vi "TS-70.vi"() -> ()   [LabVIEW 2018]
uses:
  <vilib>/DAQmx/write.llb/DAQmx Write (Analog 1D DBL NChan 1Samp).vi
  <vilib>/DAQmx/write.llb/DAQmx Write (Digital 1D Bool NChan 1Samp 1Line).vi
  <vilib>/DAQmx/read.llb/DAQmx Read (Analog 1D DBL NChan 1Samp).vi
  <vilib>/DAQmx/read.llb/DAQmx Read (Counter 1D DBL 1Chan NSamp).vi
  <vilib>/DAQmx/read.llb/DAQmx Read (Analog 1D Wfm NChan NSamp).vi
  <vilib>/DAQmx/write.llb/DAQmx Write (Analog DBL 1Chan 1Samp).vi
  <vilib>/DAQmx/create/channels.llb/DAQmx Create Channel (AI-Voltage-Basic).vi
  <vilib>/DAQmx/create/channels.llb/DAQmx Create Channel (CI-Frequency).vi
  <vilib>/DAQmx/configure/timing.llb/DAQmx Timing (Implicit).vi
  <vilib>/DAQmx/create/channels.llb/DAQmx Create Channel (AI-Temperature-Thermocouple).vi
  <vilib>/DAQmx/create/channels.llb/DAQmx Create Channel (DO-Digital Output).vi
  <vilib>/DAQmx/miscellaneous.llb/DAQmx Fill In Error Info.vi
  <vilib>/DAQmx/create/channels.llb/DAQmx Create Channel (AO-Voltage-Basic).vi
  <vilib>/DAQmx/create/channels.llb/DAQmx Create Channel (AI-Current-Basic).vi
  <vilib>/ptbypt/NI_PtbyPt.lvlib
  <resource>/objmgr/daqmx.rc
panel:
  out "Digital Out Errors":errorcluster
  in  "Sample Data":bool
  in  "?":T1(tab)
  out "Case Temp":i32
  out "Inlet Temp":i16
  out "RPM":i16 format="%2.0f"
  out "DisGPMCal":dbl caption="Dis GPM" format="%2.0f"
  out "CaseGPM":dbl caption="Case GPM" format="%2.0f"
  out "PSI Case":dbl caption="Case PSI" format="%2.0f"
  out "PSI In":dbl caption="Inlet PSI" format="%2.0f"
  out "PSI Discharge":dbl caption="Dis PSI" format="%2.0f"
  out "Amps C - Main":dbl caption="Amps C" format="%#.2g"
  out "Amps B - Main":dbl caption="Amps B" format="%#.2g"
  out "Amps A - Main":dbl caption="Amps A" format="%#.2g"
  out "C Volts - Main":i32 caption="VAC C"
  out "B Volts - Main":i32 caption="VAC B"
  out "A Volts - Main":i32 caption="VAC A"
  out "AC Hz":i32 caption="Hz"
  in  "Sample Rate (ms)":u32=5
  out "Waveform Chart":waveform(dbl)[](graph)
  out "Output\nVoltage - Main":dbl(knob) caption="Regulator VDC" scale=0.0..10.0
  out "Amps C - Tank":u8(slide) scale=0.0..100.0
  out "Amps B - Tank":u8(slide) scale=0.0..100.0
  out "Amps A - Tank":u8(slide) scale=0.0..100.0
  out "C Volts - Ammeter":dbl caption="C VAC" format="%#_3f"
  out "B Volts - Ammeter":dbl caption="B VAC" format="%#_3f"
  out "A Volts - Ammeter":dbl caption="A VAC" format="%#_3f"
  out "AC Hz 2":dbl caption="Hz" format="%#_3f"
  out "Amps C - Ammeters":dbl caption="C Phase" format="%#.2g"
  out "Amps B - Ammeters":dbl caption="B Phase" format="%#.2g"
  out "Amps A - Ammeters":dbl caption="A Phase" format="%#.2g"
  in  "PS 1 On/Off":bool
  in  "PS 2 On/Off":bool
  out "PS1 Amps":dbl format="%#.2f"
  out "PS1 Output Gauge":dbl(knob) scale=0.0..36.0
  out "PS1 Output":dbl format="%.1f"
  in  "PS1 Scale":dbl=10.25
  in  "PS1 Offset":dbl
  out "PS1 Desired":dbl format="%.1f"
  in  "PS1 Control":dbl(slide)=28.0 min=0.0 max=36.0 step=0.5 scale=0.0..36.0
  out "PS1 Control VDC":dbl
  in  "Output Scale":dbl=1.0
  out "PS2 Amps":dbl format="%#.2f"
  out "PS2 Outpug Gauge":dbl(knob) scale=0.0..36.0
  out "PS2 Output":dbl format="%.1f"
  in  "PS2 Scale":dbl=10.07
  in  "PS2 Offset":dbl
  out "PS2 Desired":dbl format="%.1f"
  in  "PS2 Control":dbl(slide)=28.0 min=0.0 max=36.0 step=0.5 scale=0.0..36.0
  out "PS2 Control VDC":dbl
  in  "Output Scale 2":dbl=1.0
  out "Temp Setting\nError":bool
  out "Output\nVoltage - Temp":dbl(knob) scale=0.0..10.0
  in  "Low Temp":i16
  in  "High Temp":i16
  out "Case Temp 2":i16(slide) scale=-25.0..250.0
  out "Inlet Temp 2":i16(slide) scale=-25.0..250.0
  in  "Relay 4":bool
  in  "Timed Relay":bool
  out "Boolean":bool
  in  "Off Time":dbl=1.0
  in  "On Time":dbl=2.0
  in  "RPM Offset":dbl format="%#_13g"
  in  "RPM Scale":dbl=1.0 format="%#_13g"
  out "RPM":i16 caption="Indicated"
  in  "CaseGPM Offset":dbl format="%#_13g"
  in  "CaseGPM Scale":dbl=1.0 format="%#_13g"
  out "CaseGPMCal":dbl caption="Indicated"
  in  "DisGPM Offset":dbl format="%#_13g"
  in  "DisGPM Scale":dbl=10.0 format="%#_13g"
  out "DisGPM":dbl caption="Indicated"
  in  "CasePSI Offset":dbl format="%#_13g"
  in  "CasePSI Scale":dbl=200.0 format="%#_13g"
  out "CasePSI":dbl caption="Indicated"
  in  "InPSI Offset":dbl format="%#_13g"
  in  "InPSI Scale":dbl=100.0 format="%#_13g"
  out "InPSI Ind":dbl caption="Indicated"
  in  "DisPSI Offset":dbl format="%#_13g"
  in  "DisPSI Scale":dbl=1000.0 format="%#_13g"
  out "DisPSI - Calibration":dbl caption="Indicated"
  out "AC Freq Ind":dbl caption="Indicated"
  in  "AC Freq Offset":dbl=10.0 caption="Offset" format="%#_13g"
  in  "AC Freq Scale":dbl=100.0 caption="Scale" format="%#_13g"
  out "A VAC Ind":dbl caption="Indicated"
  in  "VAC Offset A":dbl caption="Offset" format="%#_13g"
  in  "VAC Scale A":dbl=50.0 caption="Scale" format="%#_13g"
  out "B Volts - Calibration":dbl caption="Indicated"
  in  "Amp Offset C":dbl format="%#_13g"
  in  "Amp Offset B":dbl format="%#_13g"
  in  "Amp Offset A":dbl format="%#_13g"
  in  "Amp Scale C":dbl=9.88 format="%#_13g"
  in  "Amp Scale B":dbl=9.88 format="%#_13g"
  in  "Amp Scale A":dbl=9.88 format="%#_13g"
  in  "VAC Scale B":dbl=50.0 caption="Scale" format="%#_13g"
  in  "VAC Offset B":dbl caption="Offset" format="%#_13g"
  in  "VAC Offset C":dbl caption="Offset" format="%#_13g"
  in  "VAC Scale C":dbl=50.0 caption="Scale" format="%#_13g"
  out "C Volts - Calibration":dbl caption="Indicated"
  out "Amps A - Calibration":dbl caption="Indicated"
  out "Amps B - Calibration":dbl caption="Indicated"
  out "Amps C - Calibration":dbl caption="Indicated"
  out "error out":errorcluster
  out "Analog Out Errors":errorcluster
  # "AC Frequency"
  # "A Phase VAC"
  # "B Phase VAC"
  # "C Phase VAC"
  # "A Phase Amps"
  # "B Phase Amps"
  # "C Phase Amps"
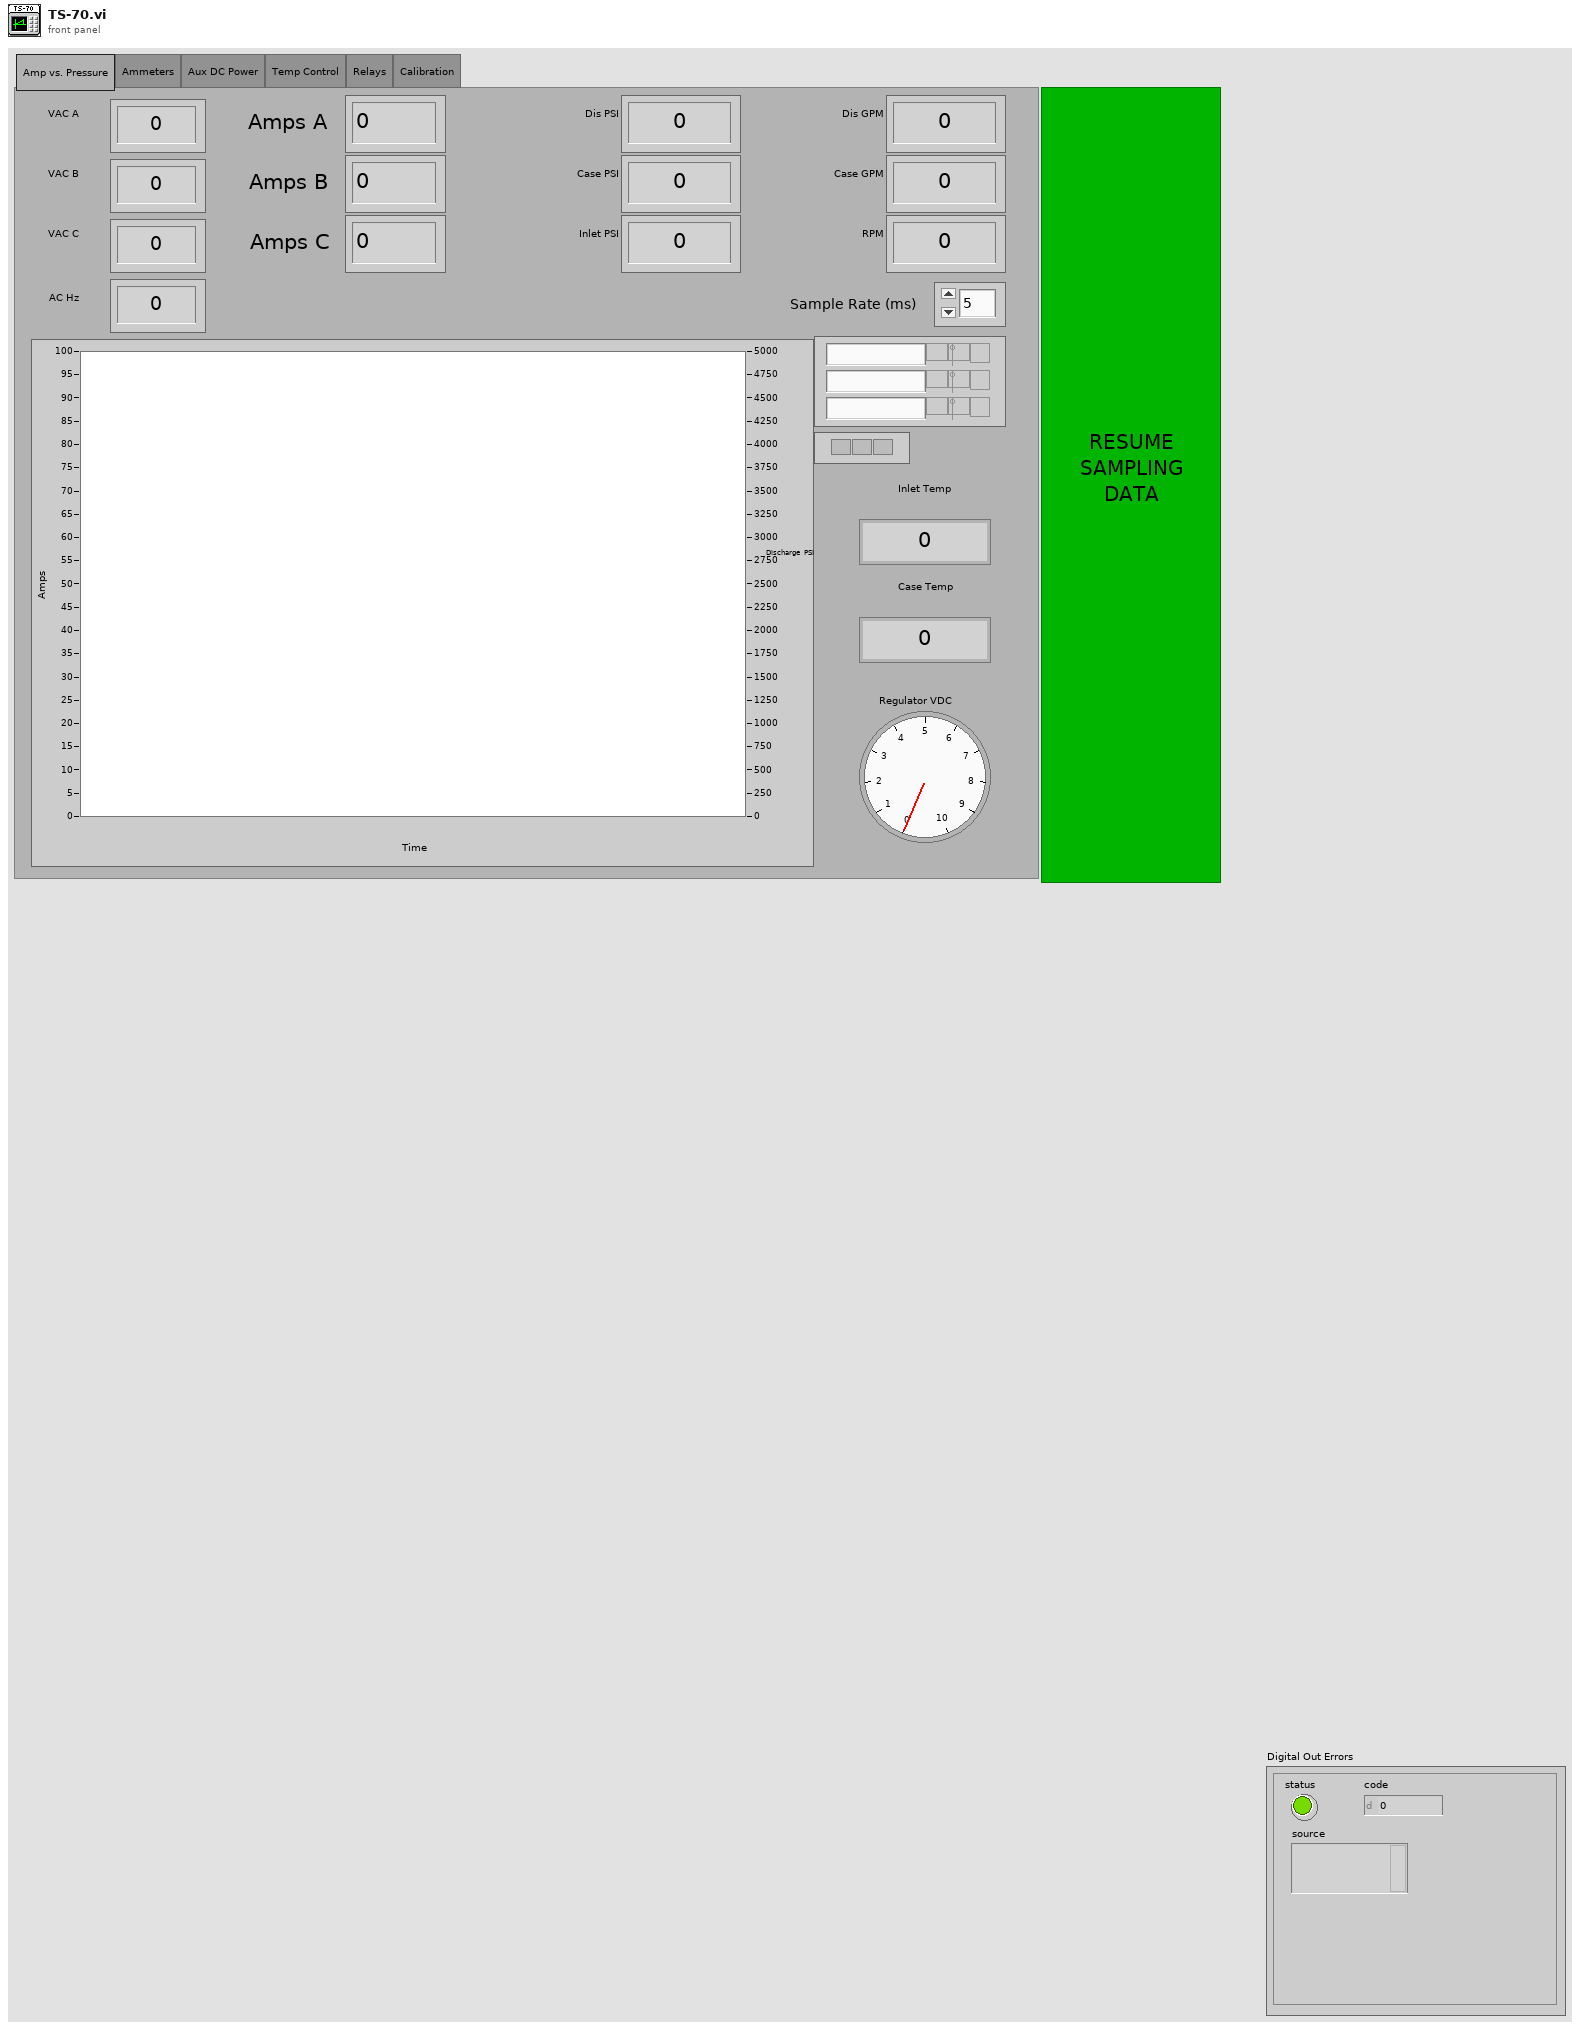
[diagram p1: front panel]
types:
  T1 = enum32{"Amp vs. Pressure", "Ammeters", "Aux DC Power", "Temp Control", "Relays", "Calibration"}
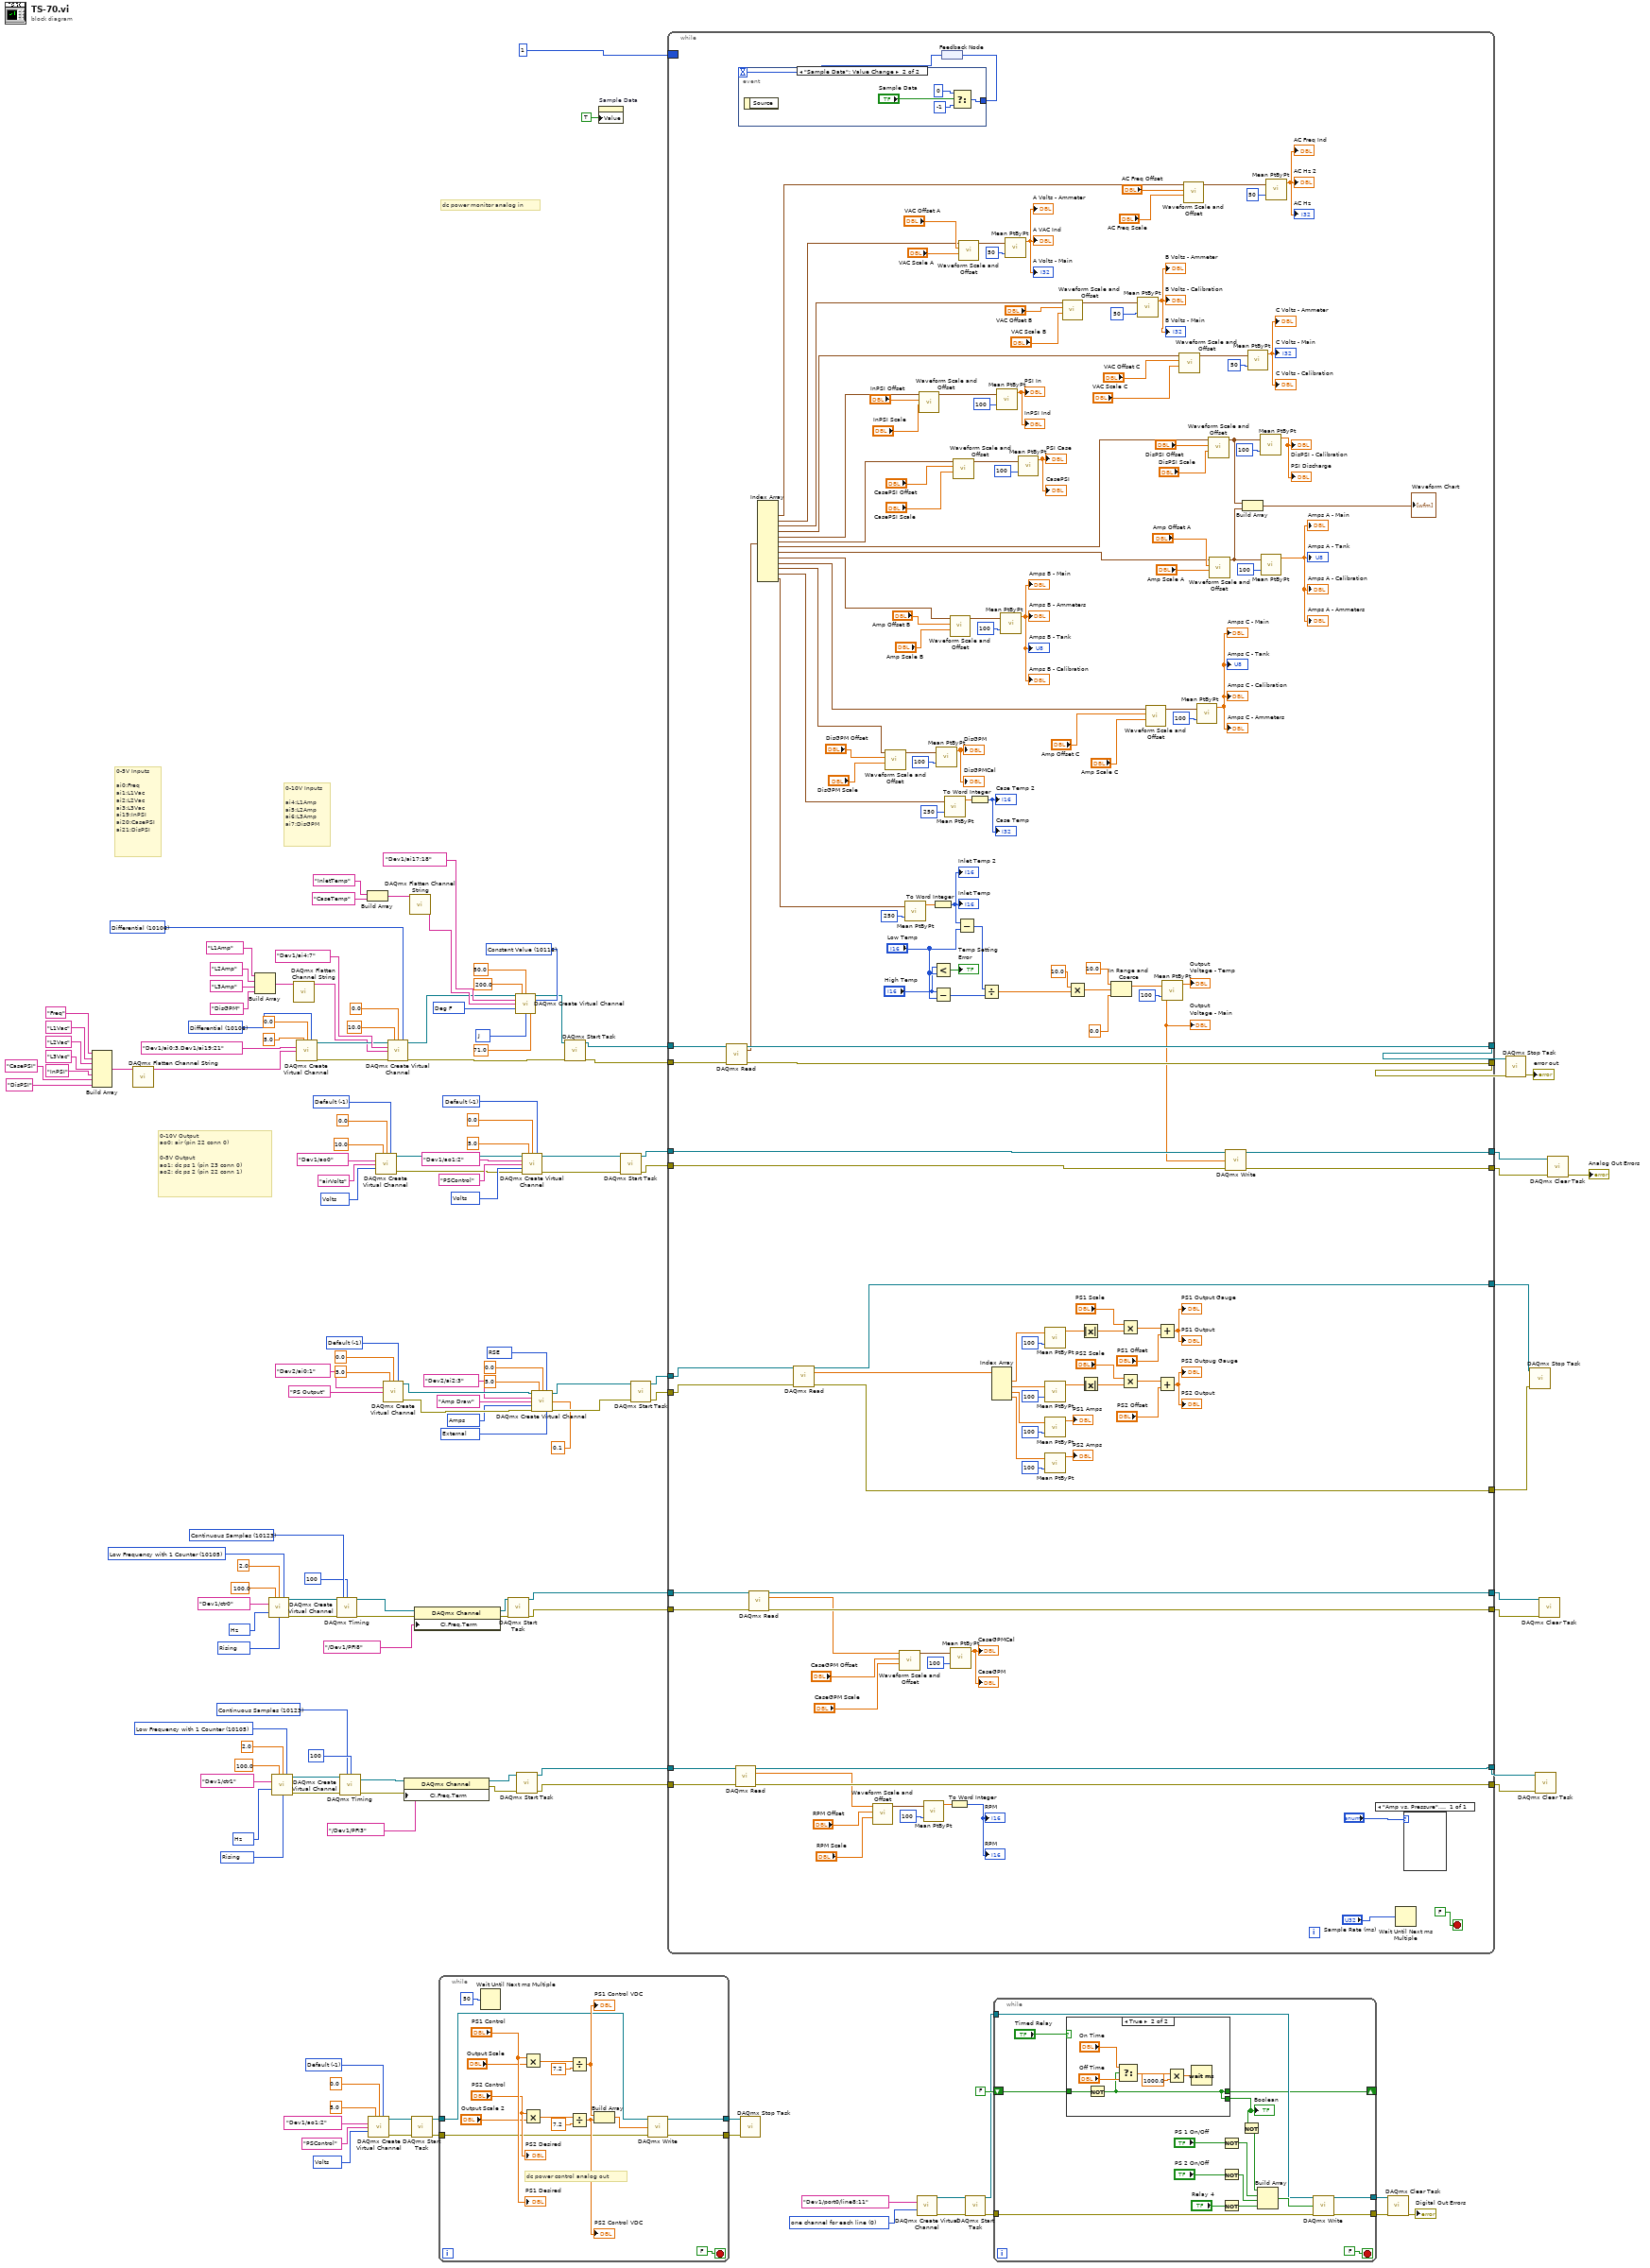
[diagram p0: block diagram]
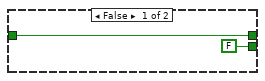
[diagram p2: hidden frame]
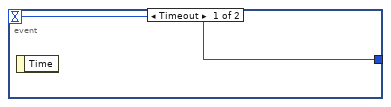
[diagram p3: hidden frame]
diagram:
  w5 = -1 items=["Default"=-1, "RSE"=10083, "Differential"=10106, "Pseudodifferential"=12529] ("output terminal configuration")
  w10 = 10348 items=["Volts"=10348, "From Custom Scale"=10065] ("units")
  w17 = 10167 items=["default"=-1, "Internal"=10200, "External"=10167] ("shunt resistor location")
  w19 = 10342 items=["Amps"=10342, "From Custom Scale"=10065] ("units")
  w22 = 10083 items=["default"=-1, "RSE"=10083, "NRSE"=10078, "Differential"=10106, "Pseudodifferential"=12529] ("input terminal configuration")
  w31 = -1 items=["Default"=-1, "RSE"=10083, "NRSE"=10078, "Differential"=10106, "Pseudodifferential"=12529] ("input terminal configuration")
  w38 = -1 items=["Default"=-1, "RSE"=10083, "Differential"=10106, "Pseudodifferential"=12529] ("output terminal configuration")
  w43 = 10348 items=["Volts"=10348, "From Custom Scale"=10065] ("units")
  w49 = -1 items=["Default"=-1, "RSE"=10083, "Differential"=10106, "Pseudodifferential"=12529] ("output terminal configuration")
  w54 = 10348 items=["Volts"=10348, "From Custom Scale"=10065] ("units")
  w61 = 0 items=["one channel for each line", "one channel for all lines"] ("line grouping")
  w68 = 10144 items=["Deg C"=10143, "Deg F"=10144, "Kelvins"=10325, "Deg R"=10145, "From Custom Scale"=10065] ("units")
  w69 = 10116 items=["Built-In"=10200, "Constant Value"=10116, "Channel"=10113] ("cjc source")
  w77 = 10072 items=["J"=10072, "K"=10073, "N"=10077, "R"=10082, "S"=10085, "T"=10086, "B"=10047, "E"=10055] ("thermocouple type")
  w92 = 10105 items=["Low Frequency with 1 Counter"=10105, "High Frequency with 2 Counters"=10157, "Large Range with 2 Counters"=10205, "Dynamic Averaging"=16065] ("measurement method")
  w91 = 10280 items=["Rising"=10280, "Falling"=10171] ("starting edge")
  w90 = 10373 items=["Hz"=10373, "Ticks"=10304, "From Custom Scale"=10065] ("units")
  w88 = 10123 items=["Finite Samples"=10178, "Continuous Samples"=10123, "Hardware Timed Single Point"=12522] ("sample mode")
  w107 = 10105 items=["Low Frequency with 1 Counter"=10105, "High Frequency with 2 Counters"=10157, "Large Range with 2 Counters"=10205, "Dynamic Averaging"=16065] ("measurement method")
  w108 = 10280 items=["Rising"=10280, "Falling"=10171] ("starting edge")
  w109 = 10373 items=["Hz"=10373, "Ticks"=10304, "From Custom Scale"=10065] ("units")
  w111 = 10123 items=["Finite Samples"=10178, "Continuous Samples"=10123, "Hardware Timed Single Point"=12522] ("sample mode")
  w142 = 10106 items=["default"=-1, "RSE"=10083, "NRSE"=10078, "Differential"=10106, "Pseudodifferential"=12529] ("input terminal configuration")
  w145 = 10106 items=["default"=-1, "RSE"=10083, "NRSE"=10078, "Differential"=10106, "Pseudodifferential"=12529] ("input terminal configuration")
  # "dc power monitor analog in"
  # "0-10V Output\nao0: air (pin 22 conn 0)\n\n0-5V Output\nao1: dc ps 1 (pin 23 conn 0)\nao2: dc ps 2 (pin 22 conn 1)"
  # "0-10V Inputs\n\nai4:L1Amp\nai5:L2Amp\nai6:L3Amp\nai7:DisGPM"
  # "0-5V Inputs\n\nai0:Freq\nai1:L1Vac\nai2:L2Vac\nai3:L3Vac\nai19:InPSI\nai20:CasePSI\nai21:DisPSI"
  n1 = Build Array("Freq", "L1Vac", "L2Vac", "L3Vac", "InPSI" ("element"), "CasePSI", "DisPSI") -> (w128:string[])
  n2 = call <vilib>:"DAQmx Flatten Channel String.vi"("names in"=w128) -> ("names out"=w127:string)  [unwired: 13 in, 1 out]
  n3 = Build Array("L1Amp", "L2Amp", "L3Amp", "DisGPM" ("element")) -> (w125:string[])
  n4 = call-poly <vilib>:"DAQmx Create Virtual Channel.vi"("maximum value"=100.0, "minimum value"=2.0, "measurement method"=w107, "counter"=tag "Dev1/ctr0", "units"=w109, "starting edge"=w108) -> ("task out"=w112:refnum<k21>, "error out"=w113:errorcluster)  [unwired: 8 in]
  n5 = call-poly <vilib>:"DAQmx Create Virtual Channel.vi"("maximum value"=100.0, "minimum value"=2.0, "measurement method"=w92, "counter"=tag "Dev1/ctr1", "units"=w90, "starting edge"=w91) -> ("task out"=w87:refnum<k21>, "error out"=w86:errorcluster)  [unwired: 8 in]
  n6 = call <vilib>:"DAQmx Flatten Channel String.vi"("names in"=w125) -> ("names out"=w121:string)  [unwired: 13 in, 1 out]
  n7 = call-poly <vilib>:"DAQmx Create Virtual Channel.vi"("maximum value"=5.0, "minimum value"=0.0, "input terminal configuration"=w145, "physical channels"=tag "Dev1/ai0:3,Dev1/ai19:21", "name to assign"=w127) -> ("task out"=w138:refnum<k21>, "error out"=w139:errorcluster)  [unwired: 9 in]
  n8 = call-poly <vilib>:"DAQmx Timing.vi"("task/channels in"=w112, "sample mode"=w111, "samples per channel"=100, "error in"=w113) -> ("task out"=w106:refnum<k21>, "error out"=w103:errorcluster)  [unwired: 10 in]
  n9 = call-poly <vilib>:"DAQmx Timing.vi"("task/channels in"=w87, "sample mode"=w88, "samples per channel"=100, "error in"=w86) -> ("task out"=w93:refnum<k21>, "error out"=w96:errorcluster)  [unwired: 10 in]
  n10 = Build Array("InletTemp", "CaseTemp") -> (w70:string[])
  n11 = call-poly <vilib>:"DAQmx Create Virtual Channel.vi"("maximum value"=5.0, "minimum value"=0.0, "output terminal configuration"=w5, "physical channels"=tag "Dev1/ao1:2", "name to assign"="PSControl", "units"=w10) -> ("task out"=w11:refnum<k21>, "error out"=w12:errorcluster)  [unwired: 8 in]
  n12 = call-poly <vilib>:"DAQmx Create Virtual Channel.vi"("maximum value"=10.0, "minimum value"=0.0, "output terminal configuration"=w49, "physical channels"=tag "Dev1/ao0", "name to assign"="airVolts", "units"=w54) -> ("task out"=w35:refnum<k21>, "error out"=w36:errorcluster)  [unwired: 8 in]
  n13 = call-poly <vilib>:"DAQmx Create Virtual Channel.vi"("maximum value"=5.0, "minimum value"=0.0, "input terminal configuration"=w31, "physical channels"=tag "Dev2/ai0:1", "name to assign"="PS Output") -> ("task out"=w28:refnum<k21>, "error out"=w25:errorcluster)  [unwired: 9 in]
  n14 = call-poly <vilib>:"DAQmx Create Virtual Channel.vi"("task in"=w138, "maximum value"=10.0, "minimum value"=0.0, "input terminal configuration"=w142, "physical channels"=tag "Dev1/ai4:7", "name to assign"=w121, "error in"=w139) -> ("task out"=w66:refnum<k21>, "error out"=w117:errorcluster)  [unwired: 7 in]
  n15 = property class="DAQmx Channel"(reference=w93, error in=w96, "CI.Freq.Term"=tag "/Dev1/PFI3") -> (reference out=w94:refnum<k21>, error out=w97:errorcluster)
  n16 = call <vilib>:"DAQmx Flatten Channel String.vi"("names in"=w70) -> ("names out"=w73:string)  [unwired: 13 in, 1 out]
  n17 = call <vilib>:"DAQmx Start Task.vi"("task/channels in"=w11, "error in"=w12) -> ("task out"=w2:refnum<k21>, "error out"=w1:errorcluster)  [unwired: 12 in]
  n18 = property class="DAQmx Channel"(reference=w106, error in=w103, "CI.Freq.Term"=tag "/Dev1/PFI8") -> (reference out=w105:refnum<k21>, error out=w102:errorcluster)
  n19 = while {
    tunnel: [w155] -> w4
    tunnel: [w154] -> w3
    tunnel: w2 -> [w153]
    tunnel: w1 -> [w152]
    stop <- FALSE stop-if-true
    # "dc power control analog out"
    n20 = Wait Until Next ms Multiple(millisecond multiple=u32 50) -> ()  [unwired: 1 out]
    n21 = Multiply(x="PS1 Control", y="Output Scale") -> (x*y=w163:dbl)
    n22 = Multiply(x="PS2 Control", y="Output Scale 2") -> (x*y=w158:dbl)
    n23 = Divide(x=w163, y=7.2) -> (x/y=w157:dbl)
    "PS1 Control VDC" <- w157
    n24 = Divide(x=w158, y=7.2) -> (x/y=w156:dbl)
    "PS2 Control VDC" <- w156
    n25 = Build Array(w157, w156) -> (w151:dbl[])
    n26 = call-poly <vilib>:"DAQmx Write.vi"("task/channels in"=w153, "data"=w151, "error in"=w152) -> ("task out"=w155:refnum<k21>, "error out"=w154:errorcluster)  [unwired: 10 in, 1 out]
    "PS1 Desired" <- "PS1 Control"
    "PS2 Desired" <- "PS2 Control"
  }
  n27 = call <vilib>:"DAQmx Start Task.vi"("task/channels in"=w105, "error in"=w102) -> ("task out"=w101:refnum<k21>, "error out"=w100:errorcluster)  [unwired: 12 in]
  n28 = call-poly <vilib>:"DAQmx Create Virtual Channel.vi"("task in"=w66, "maximum value"=200.0, "minimum value"=50.0, "physical channels"=tag "Dev1/ai17:18", "cjc source"=w69, "name to assign"=w73, "units"=w68, "thermocouple type"=w77, "cjc value"=71.0) -> ("task out"=w65:refnum<k21>)  [unwired: 5 in, 1 out]
  n29 = call <vilib>:"DAQmx Start Task.vi"("task/channels in"=w94, "error in"=w97) -> ("task out"=w82:refnum<k21>, "error out"=w81:errorcluster)  [unwired: 12 in]
  n30 = call-poly <vilib>:"DAQmx Create Virtual Channel.vi"("task in"=w35, "maximum value"=5.0, "minimum value"=0.0, "output terminal configuration"=w38, "physical channels"=tag "Dev1/ao1:2", "name to assign"="PSControl", "units"=w43, "error in"=w36) -> ("task out"=w34:refnum<k21>, "error out"=w37:errorcluster)  [unwired: 6 in]
  n31 = call-poly <vilib>:"DAQmx Create Virtual Channel.vi"("task in"=w28, "maximum value"=5.0, "minimum value"=0.0, "input terminal configuration"=w22, "physical channels"=tag "Dev2/ai2:3", "name to assign"="Amp Draw", "external shunt resistor value"=0.1, "units"=w19, "error in"=w25, "shunt resistor location"=w17) -> ("task out"=w27:refnum<k21>, "error out"=w26:errorcluster)  [unwired: 4 in]
  n32 = call <vilib>:"DAQmx Start Task.vi"("task/channels in"=w65, "error in"=w117) -> ("task out"=w120:refnum<k21>, "error out"=w148:errorcluster)  [unwired: 12 in]
  n33 = property on="Sample Data" class="Bool (strict)"("Value"=TRUE ("Sample Data")) -> ()  [unwired: 2 in, 2 out]
  n34 = call <vilib>:"DAQmx Start Task.vi"("task/channels in"=w34, "error in"=w37) -> ("task out"=w48:refnum<k21>, "error out"=w47:errorcluster)  [unwired: 12 in]
  n35 = call <vilib>:"DAQmx Start Task.vi"("task/channels in"=w27, "error in"=w26) -> ("task out"=w16:refnum<k21>, "error out"=w15:errorcluster)  [unwired: 12 in]
  n36 = while {
    tunnel: w120 -> [w315]
    tunnel: w148 -> [w267]
    tunnel: [w313] -> w137
    tunnel: [w312] -> w136
    border: 1 -> [_]
    tunnel: w101 -> [w266]
    tunnel: w100 -> [w265]
    tunnel: [w264] -> w99
    tunnel: [w263] -> w98
    tunnel: w82 -> [w262]
    tunnel: w81 -> [w261]
    tunnel: [w260] -> w80
    tunnel: [w259] -> w79
    tunnel: w48 -> [w243]
    tunnel: w47 -> [w242]
    tunnel: [w241] -> w45
    tunnel: [w240] -> w44
    tunnel: w16 -> [w169]
    tunnel: w15 -> [w168]
    tunnel: [w167] -> w14
    tunnel: [w166] -> w13
    stop <- FALSE stop-if-true
    n37 = call-poly <vilib>:"DAQmx Read.vi"("task/channels in"=w315, "error in"=w267) -> ("task out"=w312:refnum<k21>, "data"=w299:waveform(dbl)[], "error out"=w313:errorcluster)  [unwired: 11 in]
    n38 = call-poly <vilib>:"DAQmx Read.vi"("task/channels in"=w262, "error in"=w261) -> ("task out"=w260:refnum<k21>, "data"=w252:dbl[], "error out"=w259:errorcluster)  [unwired: 11 in]
    n39 = call-poly <vilib>:"DAQmx Read.vi"("task/channels in"=w266, "error in"=w265) -> ("task out"=w264:refnum<k21>, "data"=w255:dbl[], "error out"=w263:errorcluster)  [unwired: 11 in]
    n40 = Index Array(array=w299) -> (element #1=w290:waveform(dbl), element #2=w300:waveform(dbl), element #3=w294:waveform(dbl), element #4=w293:waveform(dbl), element #5=w286:waveform(dbl), element #6=w281:waveform(dbl), element #7=w289:waveform(dbl), element #8=w309:waveform(dbl), element #9=w304:waveform(dbl), element #10=w303:waveform(dbl), element #11=w258:waveform(dbl), element #12=w245:waveform(dbl), element #13=w248:waveform(dbl))  [unwired: 13 in]
    n41 = call-poly <vilib>:"DAQmx Read.vi"("task/channels in"=w169, "error in"=w168) -> ("task out"=w166:refnum<k21>, "data"=w170:dbl[], "error out"=w167:errorcluster)  [unwired: 11 in]
    n42 = call <vilib>:"Waveform Scale and Offset.vi"("scale"="RPM Scale", "offset"="RPM Offset", "waveform in"=w252) -> ("waveform out"=w222:waveform(dbl))  [unwired: 7 in, 1 out]
    n43 = call <vilib>:"Waveform Scale and Offset.vi"("scale"="DisGPM Scale", "offset"="DisGPM Offset", "waveform in"=w258) -> ("waveform out"=w224:waveform(dbl))  [unwired: 7 in, 1 out]
    n44 = call <vilib>:"Waveform Scale and Offset.vi"("scale"="CaseGPM Scale", "offset"="CaseGPM Offset", "waveform in"=w255) -> ("waveform out"=w196:waveform(dbl))  [unwired: 7 in, 1 out]
    n45 = call <vilib>:"Mean PtByPt.vi"("x"=w248, "sample length"=250) -> ("mean"=w249:dbl)  [unwired: 2 in, 1 out]
    n46 = call <vilib>:"Waveform Scale and Offset.vi"("scale"="InPSI Scale", "offset"="InPSI Offset", "waveform in"=w286) -> ("waveform out"=w201:waveform(dbl))  [unwired: 7 in, 1 out]
    n47 = call <vilib>:"Mean PtByPt.vi"("x"=w222, "sample length"=100) -> ("mean"=w221:dbl)  [unwired: 2 in, 1 out]
    n48 = To Word Integer(number=w249) -> (16bit integer=w218:i16)
    "Inlet Temp" <- w218
    "Inlet Temp 2" <- w218
    n49 = Less?(x="High Temp", y="Low Temp") -> (x < y?=→"Temp Setting\nError":bool)
    n50 = Subtract(x="High Temp", y="Low Temp") -> (x-y=w235:i16)
    n51 = call <vilib>:"Mean PtByPt.vi"("x"=w224, "sample length"=100) -> ("mean"=→"DisGPMCal" →"DisGPM":dbl)  [unwired: 2 in, 1 out]
    n52 = feedback #1() -> (w279:i32)
    n53 = event shown="[1] \"Sample Data\": Value Change" {
      selector: _ -> [_ _]
      dyn-events: _ -> [_ _]
      timeout: w279 -> [w316 _]
      tunnel: [w316 w317] -> w280
      event Timeout {
        n54 = event-data() -> ()  [unwired: 1 in, 1 out]
      }
      event "Sample Data": Value Change {
        n55 = event-data() -> ()  [unwired: 1 in, 1 out]
        n56 = Select(t=0, s="Sample Data", f=-1) -> (s? t:f=w317:i32)
      }
    }
    n57 = feedback-in #1(w280) -> ()
    n58 = call <vilib>:"Mean PtByPt.vi"("x"=w245, "sample length"=250) -> ("mean"=w246:dbl)  [unwired: 2 in, 1 out]
    n59 = To Word Integer(number=w221) -> (16bit integer=→"RPM" →"RPM":i16)
    n60 = call <vilib>:"Waveform Scale and Offset.vi"("scale"="Amp Scale B", "offset"="Amp Offset B", "waveform in"=w304) -> ("waveform out"=w210:waveform(dbl))  [unwired: 7 in, 1 out]
    n61 = call <vilib>:"Mean PtByPt.vi"("x"=w196, "sample length"=100) -> ("mean"=→"CaseGPM" →"CaseGPMCal":dbl)  [unwired: 2 in, 1 out]
    n62 = call <vilib>:"Waveform Scale and Offset.vi"("scale"="CasePSI Scale", "offset"="CasePSI Offset", "waveform in"=w281) -> ("waveform out"=w199:waveform(dbl))  [unwired: 7 in, 1 out]
    n63 = Subtract(x=w218, y="Low Temp") -> (x-y=w234:i16)
    n64 = call <vilib>:"Waveform Scale and Offset.vi"("scale"="VAC Scale A", "offset"="VAC Offset A", "waveform in"=w300) -> ("waveform out"=w278:waveform(dbl))  [unwired: 7 in, 1 out]
    n65 = To Word Integer(number=w246) -> (16bit integer=→"Case Temp" →"Case Temp 2":i16)
    n66 = Divide(x=w234, y=w235) -> (x/y=w236:dbl)
    n67 = Index Array(array=w170) -> (element #1=w174:dbl, element #2=w173:dbl, element #3=w172:dbl, element #4=w171:dbl)  [unwired: 4 in]
    n68 = call <vilib>:"Mean PtByPt.vi"("x"=w201, "sample length"=100) -> ("mean"=→"InPSI Ind" →"PSI In":dbl)  [unwired: 2 in, 1 out]
    n69 = call <vilib>:"Mean PtByPt.vi"("x"=w210, "sample length"=100) -> ("mean"=→"Amps B - Ammeters" →"Amps B - Tank" →"Amps B - Calibration" →"Amps B - Main":dbl)  [unwired: 2 in, 1 out]
    n70 = call <vilib>:"Mean PtByPt.vi"("x"=w278, "sample length"=50) -> ("mean"=→"A VAC Ind" →"A Volts - Ammeter" →"A Volts - Main":dbl)  [unwired: 2 in, 1 out]
    n71 = call <vilib>:"Mean PtByPt.vi"("x"=w199, "sample length"=100) -> ("mean"=→"CasePSI" →"PSI Case":dbl)  [unwired: 2 in, 1 out]
    n72 = call <vilib>:"Mean PtByPt.vi"("x"=w174, "sample length"=100) -> ("mean"=w187:dbl)  [unwired: 2 in, 1 out]
    n73 = call <vilib>:"Mean PtByPt.vi"("x"=w173, "sample length"=100) -> ("mean"=w183:dbl)  [unwired: 2 in, 1 out]
    n74 = call <vilib>:"Mean PtByPt.vi"("x"=w172, "sample length"=100) -> ("mean"=→"PS1 Amps":dbl)  [unwired: 2 in, 1 out]
    n75 = call <vilib>:"Mean PtByPt.vi"("x"=w171, "sample length"=100) -> ("mean"=→"PS2 Amps":dbl)  [unwired: 2 in, 1 out]
    n76 = call <vilib>:"Waveform Scale and Offset.vi"("scale"="VAC Scale B", "offset"="VAC Offset B", "waveform in"=w294) -> ("waveform out"=w274:waveform(dbl))  [unwired: 7 in, 1 out]
    n77 = Multiply(x=10.0, y=w236) -> (x*y=w204:dbl)
    n78 = Absolute Value(x=w187) -> (abs(x)=w186:dbl)
    n79 = Absolute Value(x=w183) -> (abs(x)=w182:dbl)
    n80 = In Range and Coerce(upper limit=10.0, x=w204, lower limit=0.0) -> (coerced(x)=w230:dbl)  [unwired: 1 out]
    n81 = Multiply(x="PS1 Scale", y=w186) -> (x*y=w185:dbl)
    n82 = Multiply(x="PS2 Scale", y=w182) -> (x*y=w181:dbl)
    n83 = call <vilib>:"Mean PtByPt.vi"("x"=w274, "sample length"=50) -> ("mean"=→"B Volts - Calibration" →"B Volts - Ammeter" →"B Volts - Main":dbl)  [unwired: 2 in, 1 out]
    n84 = call <vilib>:"Waveform Scale and Offset.vi"("scale"="Amp Scale C", "offset"="Amp Offset C", "waveform in"=w303) -> ("waveform out"=w213:waveform(dbl))  [unwired: 7 in, 1 out]
    n85 = Add(x=w185, y="PS1 Offset") -> (x+y=→"PS1 Output Gauge" →"PS1 Output":dbl)
    n86 = Add(x=w181, y="PS2 Offset") -> (x+y=→"PS2 Outpug Gauge" →"PS2 Output":dbl)
    n87 = call <vilib>:"Mean PtByPt.vi"("x"=w230, "sample length"=100) -> ("mean"=w229:dbl)  [unwired: 2 in, 1 out]
    "Output\nVoltage - Temp" <- w229
    "Output\nVoltage - Main" <- w229
    n88 = call <vilib>:"Waveform Scale and Offset.vi"("scale"="VAC Scale C", "offset"="VAC Offset C", "waveform in"=w293) -> ("waveform out"=w273:waveform(dbl))  [unwired: 7 in, 1 out]
    n89 = call <vilib>:"Waveform Scale and Offset.vi"("scale"="AC Freq Scale", "offset"="AC Freq Offset", "waveform in"=w290) -> ("waveform out"=w270:waveform(dbl))  [unwired: 7 in, 1 out]
    n90 = call <vilib>:"Mean PtByPt.vi"("x"=w213, "sample length"=100) -> ("mean"=→"Amps C - Ammeters" →"Amps C - Tank" →"Amps C - Calibration" →"Amps C - Main":dbl)  [unwired: 2 in, 1 out]
    n91 = call <vilib>:"Waveform Scale and Offset.vi"("scale"="DisPSI Scale", "offset"="DisPSI Offset", "waveform in"=w289) -> ("waveform out"=w205:waveform(dbl))  [unwired: 7 in, 1 out]
    n92 = call <vilib>:"Waveform Scale and Offset.vi"("scale"="Amp Scale A", "offset"="Amp Offset A", "waveform in"=w309) -> ("waveform out"=w207:waveform(dbl))  [unwired: 7 in, 1 out]
    n93 = call-poly <vilib>:"DAQmx Write.vi"("task/channels in"=w243, "data"=w229, "error in"=w242) -> ("task out"=w241:refnum<k21>, "error out"=w240:errorcluster)  [unwired: 10 in, 1 out]
    n94 = Build Array(w205, w207) -> (→"Waveform Chart":waveform(dbl)[])
    n95 = call <vilib>:"Mean PtByPt.vi"("x"=w273, "sample length"=50) -> ("mean"=→"C Volts - Calibration" →"C Volts - Ammeter" →"C Volts - Main":dbl)  [unwired: 2 in, 1 out]
    n96 = call <vilib>:"Mean PtByPt.vi"("x"=w205, "sample length"=100) -> ("mean"=→"PSI Discharge" →"DisPSI - Calibration":dbl)  [unwired: 2 in, 1 out]
    n97 = call <vilib>:"Mean PtByPt.vi"("x"=w207, "sample length"=100) -> ("mean"=→"Amps A - Ammeters" →"Amps A - Tank" →"Amps A - Calibration" →"Amps A - Main":dbl)  [unwired: 2 in, 1 out]
    n98 = call <vilib>:"Mean PtByPt.vi"("x"=w270, "sample length"=50) -> ("mean"=→"AC Freq Ind" →"AC Hz 2" →"AC Hz":dbl)  [unwired: 2 in, 1 out]
    n99 = Wait Until Next ms Multiple(millisecond multiple="Sample Rate (ms)") -> ()  [unwired: 1 out]
    n100 = case shown="\"Amp vs. Pressure\", Default" "?" {
      frame "Amp vs. Pressure", Default {
      }
    }
  }
  n101 = call <vilib>:"DAQmx Stop Task.vi"("task/channels in"=w4, "error in"=w3) -> ()  [unwired: 12 in, 2 out]
  n102 = call-poly <vilib>:"DAQmx Create Virtual Channel.vi"("lines"=tag "Dev1/port0/line8:11", "line grouping"=w61) -> ("task out"=w64:refnum<k21>, "error out"=w63:errorcluster)  [unwired: 12 in]
  n103 = call <vilib>:"DAQmx Start Task.vi"("task/channels in"=w64, "error in"=w63) -> ("task out"=w58:refnum<k21>, "error out"=w57:errorcluster)  [unwired: 12 in]
  n104 = while {
    shift-right: [w327] -> _
    shift-left: FALSE -> [w336]
    tunnel: w58 -> [w331]
    tunnel: w57 -> [w330]
    tunnel: [w328] -> w56
    tunnel: [w329] -> w55
    stop <- FALSE stop-if-true
    n105 = case shown="True" "Timed Relay" {
      tunnel: w336 -> [w339 w346]
      tunnel: [w339 w340] -> w327
      tunnel: [FALSE w340] -> w325
      frame False {
      }
      frame True {
        n106 = Not(x=w346) -> (.not. x?=w340:bool)
        n107 = Select(t="On Time", s=w340, f="Off Time") -> (s? t:f=w345:dbl)
        n108 = Multiply(x=w345, y=1000.0) -> (x*y=w341:dbl)
        n109 = Wait (ms)(milliseconds to wait=w341) -> ()  [unwired: 1 out]
      }
    }
    "Boolean" <- w325
    n110 = Not(x="PS 1 On/Off") -> (.not. x?=w324:bool)
    n111 = Not(x="PS 2 On/Off") -> (.not. x?=w323:bool)
    n112 = Not(x="Relay 4") -> (.not. x?=w322:bool)
    n113 = Not(x=w325) -> (.not. x?=w321:bool)
    n114 = Build Array(w321, w324, w323, w322) -> (w335:bool[])
    n115 = call-poly <vilib>:"DAQmx Write.vi"("task/channels in"=w331, "data"=w335, "error in"=w330) -> ("task out"=w328:refnum<k21>, "error out"=w329:errorcluster)  [unwired: 10 in, 1 out]
  }
  n116 = call <vilib>:"DAQmx Clear Task.vi"("task in"=w56, "error in"=w55) -> ("error out"=→"Digital Out Errors":errorcluster)  [unwired: 13 in]
  n117 = call <vilib>:"DAQmx Stop Task.vi"("task/channels in"=w136, "error in"=w137) -> ("error out"=→"error out":errorcluster)  [unwired: 12 in, 1 out]
  n118 = call <vilib>:"DAQmx Stop Task.vi"("task/channels in"=w13, "error in"=w14) -> ()  [unwired: 12 in, 2 out]
  n119 = call <vilib>:"DAQmx Clear Task.vi"("task in"=w80, "error in"=w79) -> ()  [unwired: 13 in, 1 out]
  n120 = call <vilib>:"DAQmx Clear Task.vi"("task in"=w99, "error in"=w98) -> ()  [unwired: 13 in, 1 out]
  n121 = call <vilib>:"DAQmx Clear Task.vi"("task in"=w45, "error in"=w44) -> ("error out"=→"Analog Out Errors":errorcluster)  [unwired: 13 in]
